vi "GetStrListFrom2DListCtrl.vi"(10 "include index?":bool, 11 "ref 2D list in":refnum<vi>) -> (2 "result":string[][](array[string]), 3 "ref 2D list out":refnum<vi>)   [LabVIEW 2018, in "Library-Ctrl.lvlib"]
uses:
  Library-Ctrl.lvlib
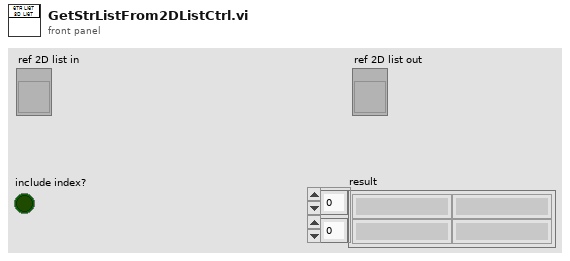
[diagram p1: front panel]
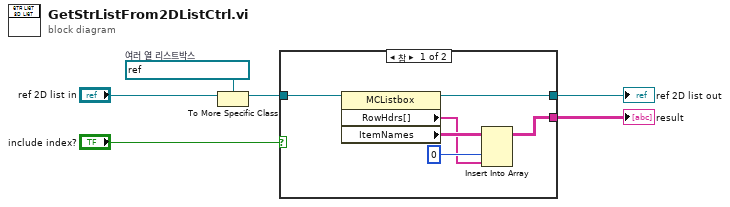
[diagram p0: block diagram]
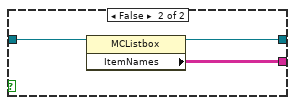
[diagram p2: hidden frame]
diagram:
  w3 = refnum<vi> refnum  # 여러 열 리스트박스
  n1 = To More Specific Class(target class=w3, reference="ref 2D list in") -> (specific class reference=w1:refnum<vi>)  [unwired: 1 in, 1 out]
  n2 = case shown="참" "include index?" {
    tunnel: w1 -> [w12 w15]
    tunnel: [w7 w14] -> w6
    tunnel: [w11 w13] -> w5
    frame True {
      n3 = property class="MCListbox"(reference=w12) -> (reference out=w11:refnum<vi>, "RowHdrs[]"=w8:string[], "ItemNames"=w10:string[][])  [unwired: 1 in, 1 out]
      n4 = Insert Into Array(array=w10, index (col)=0 ("비활성화된 인덱스 (열)"), new element=w8) -> (w7:string[][])  [unwired: 1 in]
    }
    frame False {
      n5 = property class="MCListbox"(reference=w15) -> (reference out=w13:refnum<vi>, "ItemNames"=w14:string[][])  [unwired: 1 in, 1 out]
    }
  }
  "result" <- w6
  "ref 2D list out" <- w5
